vi "Move to position.vi"(8 "error in (no error)":errorcluster, 10 "Position":dbl, 11 "Motor in":refnum<class "Motor.lvclass">) -> (0 "error out":errorcluster, 3 "Motor out":refnum<class "Motor.lvclass">)   [LabVIEW 2019, in "Motor.lvclass"]
uses:
  Motor.lvclass
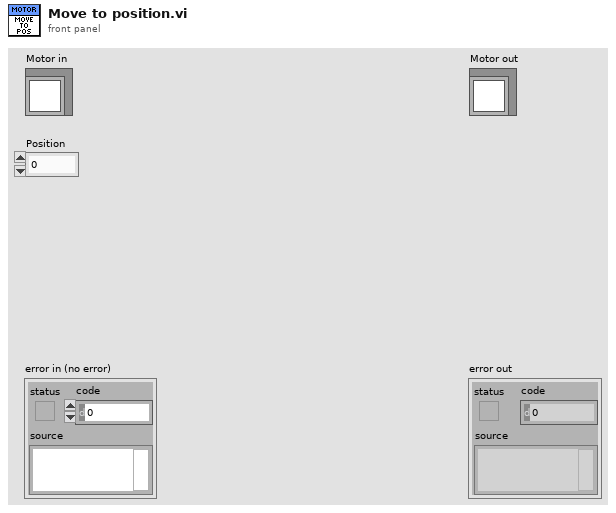
[diagram p1: front panel]
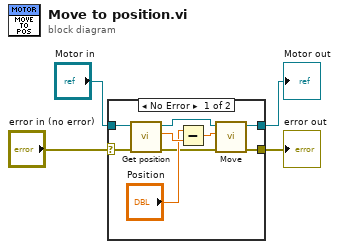
[diagram p0: block diagram]
diagram:
  n1 = case shown="No Error" "error in (no error)" {
    selector: "error in (no error)" -> [w8 w15]
    tunnel: [w7 w15] -> w3
    tunnel: [w6 w14] -> w1
    tunnel: "Motor in" -> [w13 w14]
    frame No Error {
      n2 = call-dynamic "Get position.vi"("error in (no error)"=w8, "Motor in"=w13) -> ("error out"=w9:errorcluster, "Position (rev)"=w12:dbl, "Motor out"=w5:refnum<class "Motor.lvclass">)  [unwired: 7 in]
      n3 = Subtract(x="Position", y=w12) -> (x-y=w10:dbl)
      n4 = call-dynamic "Move.vi"("error in (no error)"=w9, "Amount (rev)"=w10, "Motor in"=w5) -> ("error out"=w7:errorcluster, "Motor out"=w6:refnum<class "Motor.lvclass">)  [unwired: 7 in]
    }
    frame Error {
    }
  }
  "error out" <- w3
  "Motor out" <- w1
